vi "Destroy Panel GUI Manager.vi"(8 "error in (no error)":errorcluster, 11 "Panel GUI Manager in":refnum<class "Panel GUI Manager.lvclass">) -> (0 "error out":errorcluster, 3 "Panel GUI Manager out":refnum<class "Panel GUI Manager.lvclass">)   [LabVIEW 2015, in "Panel GUI Manager.lvclass"]
uses:
  Panel GUI Manager.lvclass
  Panel GUI Manager.lvclass/Panel GUI Manager.ctl
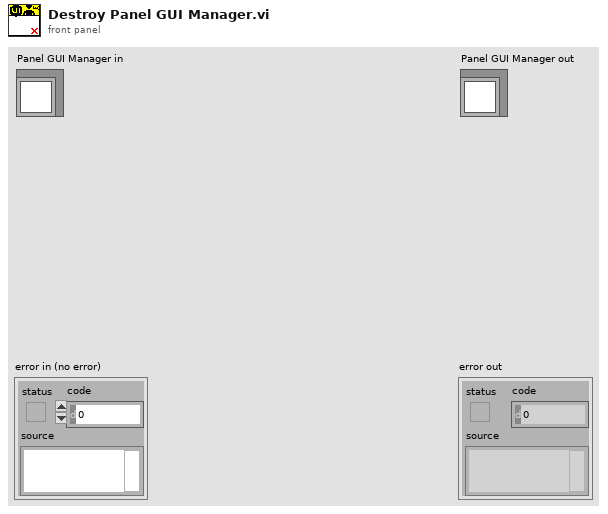
[diagram p1: front panel]
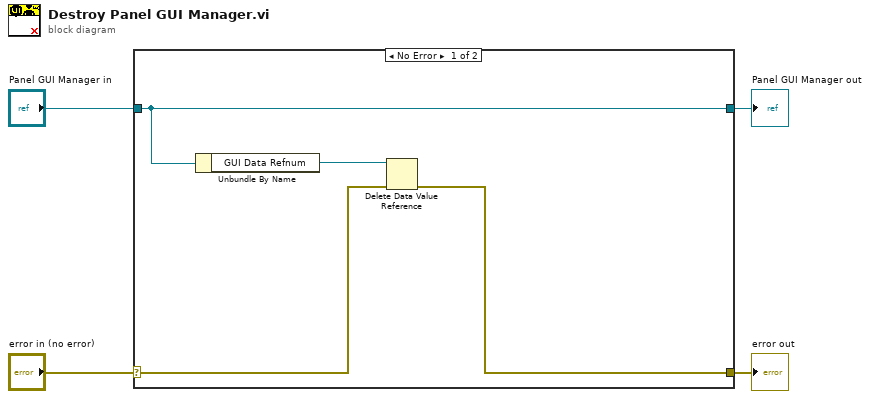
[diagram p0: block diagram]
diagram:
  n1 = case shown="No Error" "error in (no error)" {
    selector: "error in (no error)" -> [w6 w10]
    tunnel: [w5 w10] -> w3
    tunnel: [w8 w9] -> w1
    tunnel: "Panel GUI Manager in" -> [w8 w9]
    frame No Error {
      n2 = Unbundle By Name(w8) -> ("GUI Data Refnum"=w7:refnum<data-value>)
      n3 = Delete Data Value Reference(data value reference=w7, error in=w6) -> (error out=w5:errorcluster)  [unwired: 1 out]
    }
    frame Error {
    }
  }
  "error out" <- w3
  "Panel GUI Manager out" <- w1
